vi "ActionVIOnSave.vi"(8 "error in (no error)":errorcluster, 11 "Device Item Ref in":T1 format="%.0x") -> (0 "error out":errorcluster, 3 "Device Item Ref out":T1 format="%.0x")   [LabVIEW 2020, in "Routing and Faulting System Explorer.lvlib"]
uses:
  Routing and Faulting System Explorer.lvlib
  <vilib>/NI VeriStand/Custom Device API/Custom Device Item Ref.ctl
  <vilib>/NI VeriStand/Custom Device API/Custom Device API.lvlib
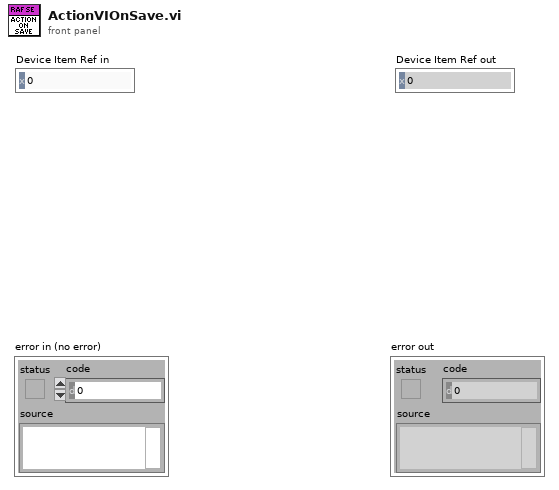
[diagram p1: front panel]
types:
  T1 = typedef "Custom Device API.lvlib/Custom Device Item Ref.ctl" = u64
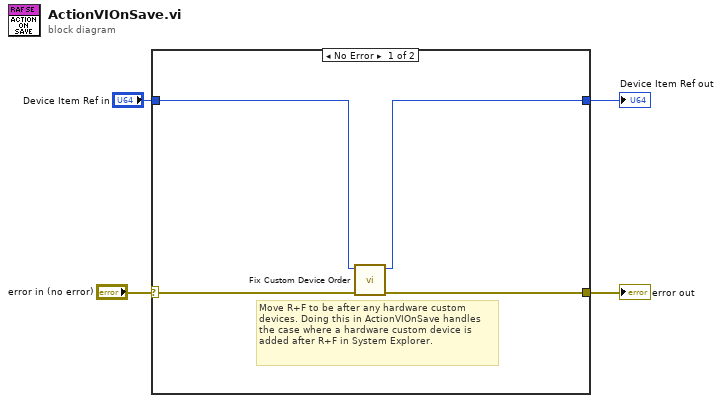
[diagram p0: block diagram]
diagram:
  n1 = case shown="No Error" "error in (no error)" {
    selector: "error in (no error)" -> [w8 w10]
    tunnel: [w7 w10] -> w3
    tunnel: "Device Item Ref in" -> [w6 w9]
    tunnel: [w5 w9] -> w1
    frame No Error {
      # "Move R+F to be after any hardware custom devices. Doing this in ActionVIOnSave handles the case where a hardware custom device is added after R+F in System Explorer."
      n2 = call "Fix Custom Device Order.vi"("error in"=w8, "Device Item Ref in"=w6) -> ("error out"=w7:errorcluster, "Device Item Ref out"=w5:T1)  [unwired: 8 in]
    }
    frame Error {
    }
  }
  "error out" <- w3
  "Device Item Ref out" <- w1
